vi "GetFrontPanel.vi"(8 "Error In":errorcluster, 11 "reference in":refnum<class "TemplateGUI.lvclass">) -> (0 "Error Out":errorcluster, 2 "FrontPanel":refnum<class "FrontPanelControl.lvclass">, 3 "reference in":refnum<class "TemplateGUI.lvclass">)   [LabVIEW 2021, in "TemplateGUI.lvlib" / "TemplateGUI.lvclass"]
uses:
  TemplateGUI.lvclass
  .Externals/Library_UserInterface_FrontPanelControl/FrontPanelControl/FrontPanelControl.lvclass
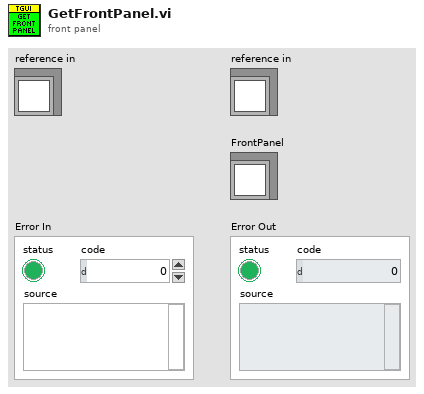
[diagram p1: front panel]
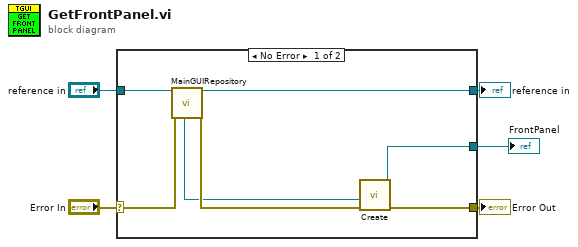
[diagram p0: block diagram]
diagram:
  n1 = case shown="No Error" "Error In" {
    selector: "Error In" -> [w10 w14]
    tunnel: [w8 w14] -> w4
    tunnel: [w11 w13] -> w2
    tunnel: "reference in" -> [w12 w13]
    tunnel: [w6 _] -> w1
    frame No Error {
      n2 = call "MainGUIRepository.vi"("reference in"=w12, "Error In"=w10) -> ("ProcessViRef"=w7:refnum<vi>, "reference out"=w11:refnum<class "TemplateGUI.lvclass">, "Error Out"=w9:errorcluster)  [unwired: 10 in, 5 out]
      n3 = call "Create.vi"("Error In"=w9, "VIRef"=w7) -> ("Error Out"=w8:errorcluster, "object out"=w6:refnum<class "FrontPanelControl.lvclass">)  [unwired: 8 in]
    }
    frame Error {
    }
  }
  "Error Out" <- w4
  "reference in" <- w2
  "FrontPanel" <- w1
